vi "Autonomous Independent.vi"   [LabVIEW 2015]
doc: "This VI is called when autonomous begins, and will automatically be terminated when autonomous ends. You can carry out timed or sensor driven robot movement independently without needing to return to the caller."
uses:
  <vilib>/Rock Robotics/WPI/Utilities/WPI_GetSetVariantRefNum.vi
  <vilib>/Rock Robotics/Network Tables/NT Read String.vi
  <vilib>/Rock Robotics/Network Tables/NT Read Number.vi
  <vilib>/Rock Robotics/Network Tables/NT Write Numeric Array.vi
  <vilib>/Rock Robotics/Network Tables/NT Read Boolean.vi
panel:
  # "Be sure to right-click and choose Data Operations>>Make Current Value default if you want to save the array values with the VI"
types:
  T1 = typedef "WPI_JoystickDevRef.ctl" = cluster{"Device":T2}
  T2 = typedef "WPI_JoystickDeviceEnum.ctl" = enum16{"USB 0", "USB 1", "USB 2", "USB 3", "USB 4", "USB 5"}
  T3 = typedef "WPI_EncoderDevRef.ctl" = cluster{"DevStatus":errorcluster, "EncoderIndex":T4, "CounterIndex":T5, "DistancePerCount":dbl, "Decoding Type":T6}
  T4 = typedef "FPGA_EncoderIdx.ctl" = enum8{"Enc 0", "Enc 1", "Enc 2", "Enc 3", "Enc 4", "Enc 5", "Enc 6", "Enc 7", "Invalid"}
  T5 = typedef "FPGA_CounterCtrSystemIndex.ctl" = enum8{"Ctr 0", "Ctr 1", "Ctr 2", "Ctr 3", "Ctr 4", "Ctr 5", "Ctr 6", "Ctr 7", "Invalid"}
  T6 = typedef "WPI_EncoderType.ctl" = enum16{"1x", "2x", "4x"}
  T7 = typedef "WPI_MotorControlDeviceRef.ctl" = cluster{"DeviceStatus":errorcluster, "Type":T8, "PWM":cluster{"PWM Channel":T9, "DeadBand":T10}, "CAN":cluster{"Device Number":u8, "Control Mode":T11, "Semaphore":T12, "Max Vout":dbl, "TalonSRX Control Mode":T13}, "Invert":bool}
  T8 = typedef "WPI_MotorControlType.ctl" = enum16{"PWM", "CAN", "CANTalonSRX"}
  T9 = typedef "FPGA_DIOPWMChannel.ctl" = enum8{"PWM 0", "PWM 1", "PWM 2", "PWM 3", "PWM 4", "PWM 5", "PWM 6", "PWM 7", "PWM 8", "PWM 9", "PWM MXP 0", "PWM MXP 1", "PWM MXP 2", "PWM MXP 3", "PWM MXP 4", "PWM MXP 5", "PWM MXP 6", "PWM MXP 7", "PWM MXP 8", "PWM MXP 9", "Invalid"}
  T10 = typedef "WPI_PWMDeadband.ctl" = cluster{"Name":string, "maxPositivePwm":i32, "minPositivePwm":i32, "centerPwm":i32, "maxNegativePwm":i32, "minNegativePwm":i32, "angularRange":u16}
  T11 = typedef "WPI_CANJaguar_ControlMode.ctl" = enum8{"Percent VBus", "Current", "Speed", "Position", "Voltage"}
  T12 = typedef "Semaphore RefNum" = refnum<k1>
  T13 = typedef "WPI_CANTalonSRX_APIControlMode.ctl" = enum8{"Percent VBus", "Speed", "Position", "Slave", "Unchanged / Invalid", "Voltage Compensation", "Current", "Motion Profile"}
  T14 = typedef "WPI_GyroDevRef.ctl" = cluster{"DevStatus":errorcluster, "Analog Channel":T15, "Offset":dbl, "Gain (VoltsPerDegree/Second)":dbl, "Gyro Type":enum16{"Analog", "XRS450"}, "Handle":i32, "SPI Bus":T16, "Device Found":bool, "Sample Rate":dbl, "Calibrate On Open":bool}
  T15 = typedef "FPGA_AIChannel.ctl" = enum8{"AI 0", "AI 1", "AI 2", "AI 3", "AI MXP 0", "AI MXP 1", "AI MXP 2", "AI MXP 3", "Invalid"}
  T16 = typedef "spi_bus.ctl" = enum16{"SPI On-Board, CS0", "SPI On-Board, CS1", "SPI On-Board, CS2", "SPI On-Board, CS3", "SPI MXP", "Invalid"}
  T17 = typedef "WPI_RobotDriveDevRef.ctl" = cluster{"DevStatus":errorcluster, "Motors[]":T7[], "Square Inputs":bool, "Max Output":dbl}
  T18 = typedef "WPI_DigitalInputDevRef.ctl" = cluster{"DevStatus":errorcluster, "DIO Channel":T19}
  T19 = typedef "FPGA_DIOChannel.ctl" = enum8{"DIO 0", "DIO 1", "DIO 2", "DIO 3", "DIO 4", "DIO 5", "DIO 6", "DIO 7", "DIO 8", "DIO 9", "DIO MXP 0", "DIO MXP 1", "DIO MXP 2", "DIO MXP 3", "DIO MXP 4", "DIO MXP 5", "DIO MXP 6", "DIO MXP 7", "DIO MXP 8", "DIO MXP 9", "DIO MXP 10", "DIO MXP 11", "DIO MXP 12", "DIO MXP 13", "DIO MXP 14", "DIO MXP 15", "Invalid"}
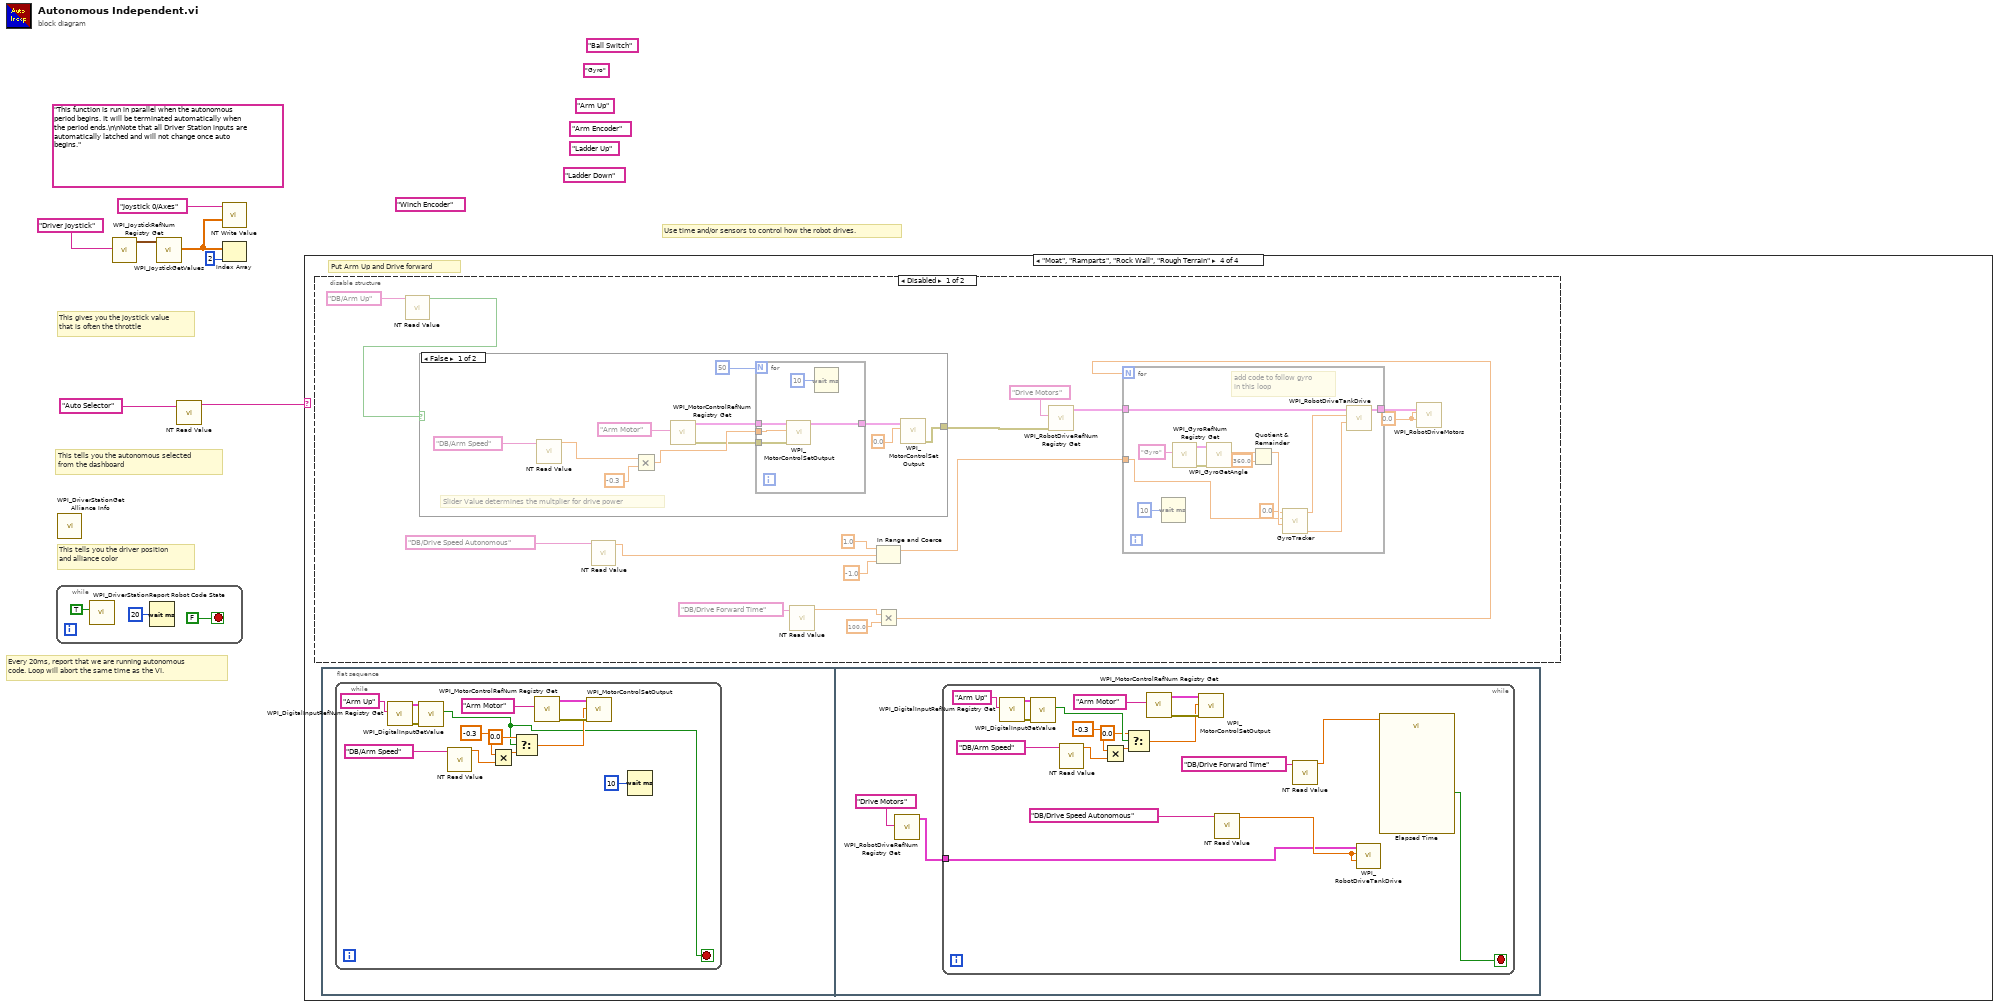
[diagram p0: block diagram]
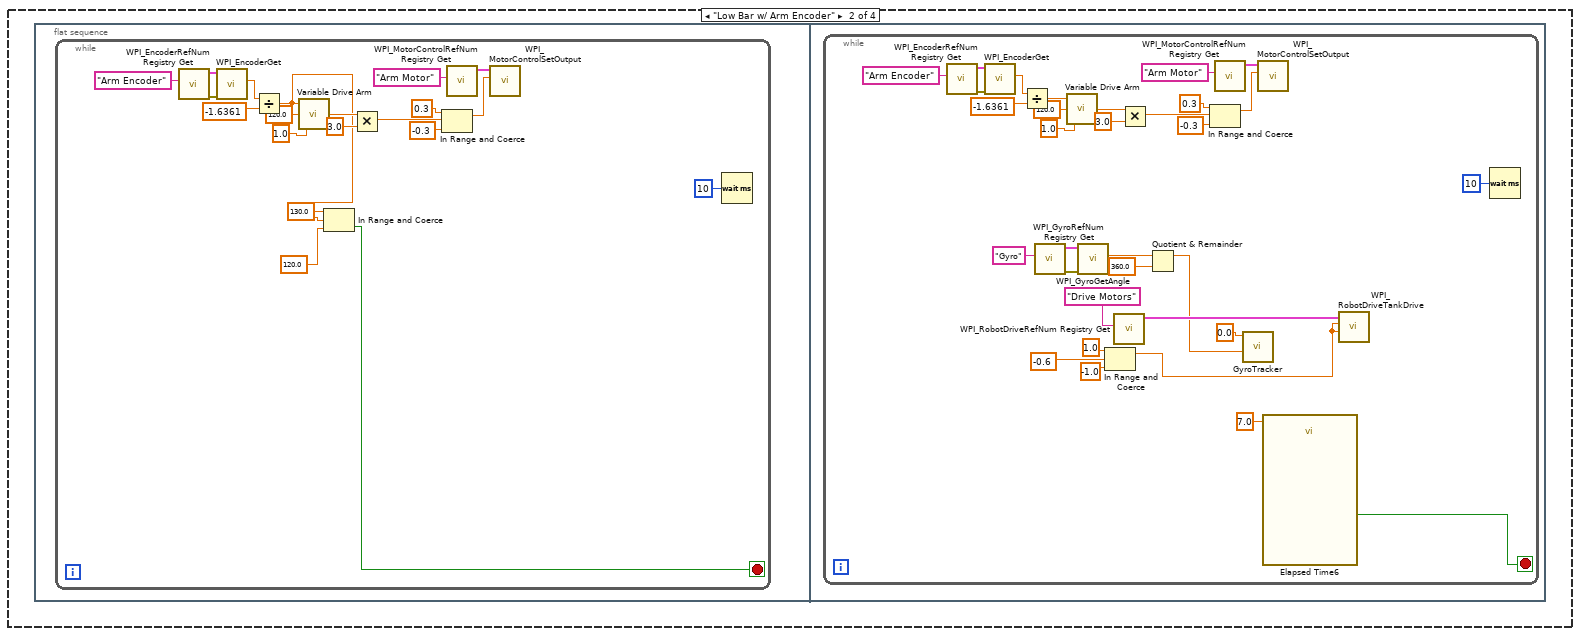
[diagram p3: hidden frame]
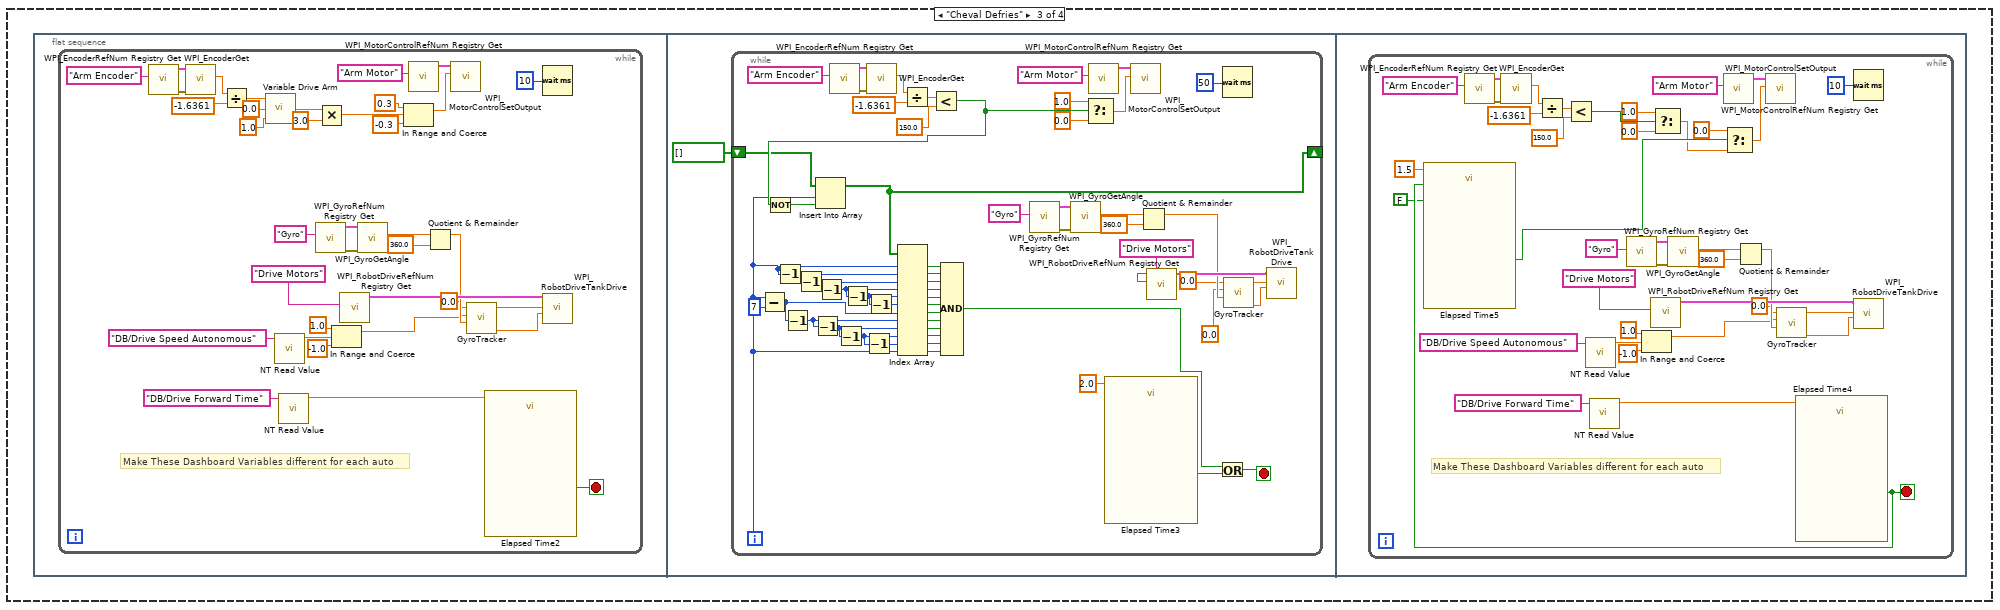
[diagram p4: hidden frame]
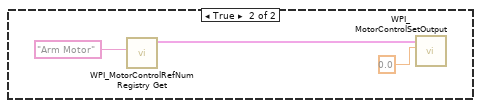
[diagram p5: hidden frame]
diagram:
  (unwired) "Arm Up" ("refnum name")
  (unwired) "Winch Encoder" ("refnum name")
  (unwired) "Ladder Down" ("refnum name")
  (unwired) "Ladder Up" ("refnum name")
  (unwired) "Arm Encoder" ("refnum name")
  (unwired) "Ball Switch" ("refnum name")
  (unwired) "Gyro" ("refnum name")
  (unwired) "This function is run in parallel when the autonomous period begins. It will be terminated automatically when the period ends.\n\nNote that all Driver Station inputs are automatically latched and will not change once auto begins."
  # "This tells you the autonomous selected\nfrom the dashboard"
  # "Every 20ms, report that we are running autonomous\ncode. Loop will abort the same time as the VI."
  # "This gives you the joystick value\nthat is often the throttle"
  # "Use time and/or sensors to control how the robot drives."
  # "This tells you the driver position\nand alliance color"
  n1 = while {
    stop <- FALSE stop-if-true
    n2 = call <vilib>:"WPI_DriverStationReport Robot Code State.vi"("Autonomous"=TRUE) -> ()  [unwired: 10 in, 1 out]
    n3 = Wait (ms)(milliseconds to wait=u32 20) -> ()  [unwired: 1 out]
  }
  n4 = call <vilib>:"WPI_DriverStationGet Alliance Info.vi"() -> ()  [unwired: 12 out]
  n5 = call <vilib>:"WPI_JoystickRefNum Registry Get.vi"("refnum name"="Driver Joystick") -> ("JoystickDevRef"=w6:T1)  [unwired: 1 in, 9 out]
  n6 = call <vilib>:"WPI_JoystickGetValues.vi"("JoystickDevRef"=w6) -> ("Axes"=w2:dbl[])  [unwired: 6 in, 4 out]
  n7 = call-poly <vilib>:"NT Read Value.vi"("Name"="Auto Selector") -> ("String"=w3:string)  [unwired: 9 in, 1 out]
  n8 = call-poly <vilib>:"NT Write Value.vi"("Numeric Array"=w2, "Name"="Joystick 0/Axes") -> ()  [unwired: 9 in, 1 out]
  n9 = Index Array(array=w2, index=2) -> ()  [unwired: 1 out]
  n10 = case shown="\"Moat\", \"Ramparts\", \"Rock Wall\", \"Rough Terrain\"" w3 {
    frame Default {
      # "You can put your main auto here, or you can right-click on the case and make any\nother frame be the default case."
      # "This is the frame that will execute if no selection is made, or if it is not recognized"
    }
    frame "Low Bar w/ Arm Encoder" {
      n11 = flat-sequence {
        frame #0 {
          n12 = while {
            stop <- w11 stop-if-true
            n13 = call <vilib>:"WPI_EncoderRefNum Registry Get.vi"("refnum name"="Arm Encoder") -> ("error out"=w24:errorcluster, "EncoderDevRef"=w25:T3)  [unwired: 9 in]
            n14 = call <vilib>:"WPI_EncoderGet.vi"("error in (no error)"=w24, "EncoderDevRef"=w25) -> ("Distance"=w26:dbl)  [unwired: 4 in, 5 out]
            n15 = Divide(x=w26, y=-1.6361 ("Arm Calibration")) -> (x/y=w14:dbl)
            n16 = call "Variable Drive Arm.vi"("Max Speed"=1.0, "Wanted Angle"=120.0, "Encoder"=w14) -> ("Motor Controller"=w18:dbl)
            n17 = In Range and Coerce(upper limit=130.0, x=w14, lower limit=120.0) -> (In Range?=w11:bool)  [unwired: 1 out]
            n18 = Multiply(x=w18, y=3.0) -> (x*y=w16:dbl)
            n19 = In Range and Coerce(upper limit=0.3, x=w16, lower limit=-0.3) -> (coerced(x)=w20:dbl)  [unwired: 1 out]
            n20 = call <vilib>:"WPI_MotorControlRefNum Registry Get.vi"("refnum name"="Arm Motor") -> ("MotorControlDevRef"=w21:T7)  [unwired: 9 in, 1 out]
            n21 = call <vilib>:"WPI_MotorControlSetOutput.vi"("Output"=w20, "MotorControlDevRef"=w21) -> ()  [unwired: 7 in, 3 out]
            n22 = Wait (ms)(milliseconds to wait=u32 10) -> ()  [unwired: 1 out]
          }
        }
        frame #1 {
          n23 = while {
            stop <- w62 stop-if-true
            n24 = call <vilib>:"WPI_EncoderRefNum Registry Get.vi"("refnum name"="Arm Encoder") -> ("error out"=w55:errorcluster, "EncoderDevRef"=w56:T3)  [unwired: 9 in]
            n25 = call <vilib>:"WPI_EncoderGet.vi"("error in (no error)"=w55, "EncoderDevRef"=w56) -> ("Distance"=w57:dbl)  [unwired: 4 in, 5 out]
            n26 = Divide(x=w57, y=-1.6361 ("Arm Calibration")) -> (x/y=w54:dbl)
            n27 = call <vilib>:"WPI_GyroRefNum Registry Get.vi"("refnum name"="Gyro") -> ("error out"=w36:errorcluster, "GyroDevRef"=w37:T14)  [unwired: 9 in]
            n28 = call "Variable Drive Arm.vi"("Max Speed"=1.0, "Wanted Angle"=120.0, "Encoder"=w54) -> ("Motor Controller"=w47:dbl)
            n29 = call <vilib>:"WPI_GyroGetAngle.vi"("error in"=w36, "GyroDevRef"=w37) -> ("Angle"=w39:dbl)  [unwired: 5 in, 4 out]
            n30 = In Range and Coerce(upper limit=1.0, x=-0.6, lower limit=-1.0) -> (coerced(x)=w33:dbl)  [unwired: 1 out]
            n31 = call <vilib>:"WPI_RobotDriveRefNum Registry Get.vi"("refnum name"="Drive Motors") -> ("RobotDriveDevRef"=w44:T17)  [unwired: 1 in, 9 out]
            n32 = Multiply(x=w47, y=3.0) -> (x*y=w45:dbl)
            n33 = Quotient & Remainder(x=w39, y=360.0) -> (x-y*floor(x/y)=w35:dbl)  [unwired: 1 out]
            n34 = In Range and Coerce(upper limit=0.3, x=w45, lower limit=-0.3) -> (coerced(x)=w50:dbl)  [unwired: 1 out]
            n35 = call <vilib>:"WPI_MotorControlRefNum Registry Get.vi"("refnum name"="Arm Motor") -> ("MotorControlDevRef"=w51:T7)  [unwired: 9 in, 1 out]
            n36 = call "GyroTracker.vi"("Gyro Angle"=w35, "Target Direction (degrees)"=0.0) -> ()  [unwired: 8 in, 2 out]
            n37 = call <vilib>:"WPI_MotorControlSetOutput.vi"("Output"=w50, "MotorControlDevRef"=w51) -> ()  [unwired: 7 in, 3 out]
            n38 = call "Elapsed Time6"("Time Target (s)"=7.0) -> ("Time has Elapsed"=w62:bool)  [unwired: 11 in, 7 out]
            n39 = call <vilib>:"WPI_RobotDriveTankDrive.vi"("Right axis value"=w33, "Left axis value"=w33, "RobotDriveDevRef"=w44) -> ()  [unwired: 6 in, 3 out]
            n40 = Wait (ms)(milliseconds to wait=u32 10) -> ()  [unwired: 1 out]
          }
        }
      }
    }
    frame "Cheval Defries" {
      n41 = flat-sequence {
        frame #0 {
          n42 = while {
            stop <- w98 stop-if-true
            # "Make These Dashboard Variables different for each auto"
            n43 = call <vilib>:"WPI_EncoderRefNum Registry Get.vi"("refnum name"="Arm Encoder") -> ("error out"=w91:errorcluster, "EncoderDevRef"=w92:T3)  [unwired: 9 in]
            n44 = call <vilib>:"WPI_EncoderGet.vi"("error in (no error)"=w91, "EncoderDevRef"=w92) -> ("Distance"=w93:dbl)  [unwired: 4 in, 5 out]
            n45 = Divide(x=w93, y=-1.6361 ("Arm Calibration")) -> (x/y=w90:dbl)
            n46 = call "Variable Drive Arm.vi"("Max Speed"=1.0, "Wanted Angle"=0.0, "Encoder"=w90) -> ("Motor Controller"=w83:dbl)
            n47 = call-poly <vilib>:"NT Read Value.vi"("Name"="DB/Drive Speed Autonomous") -> ("Numeric"=w77:dbl)  [unwired: 9 in, 1 out]
            n48 = call-poly <vilib>:"NT Read Value.vi"("Name"="DB/Drive Forward Time") -> ("Numeric"=w75:dbl)  [unwired: 9 in, 1 out]
            n49 = call <vilib>:"WPI_GyroRefNum Registry Get.vi"("refnum name"="Gyro") -> ("error out"=w66:errorcluster, "GyroDevRef"=w67:T14)  [unwired: 9 in]
            n50 = Multiply(x=w83, y=3.0) -> (x*y=w81:dbl)
            n51 = In Range and Coerce(upper limit=1.0, x=w77, lower limit=-1.0) -> (coerced(x)=w63:dbl)  [unwired: 1 out]
            n52 = call <vilib>:"WPI_RobotDriveRefNum Registry Get.vi"("refnum name"="Drive Motors") -> ("RobotDriveDevRef"=w73:T17)  [unwired: 1 in, 9 out]
            n53 = call <vilib>:"WPI_GyroGetAngle.vi"("error in"=w66, "GyroDevRef"=w67) -> ("Angle"=w69:dbl)  [unwired: 5 in, 4 out]
            n54 = In Range and Coerce(upper limit=0.3, x=w81, lower limit=-0.3) -> (coerced(x)=w86:dbl)  [unwired: 1 out]
            n55 = call <vilib>:"WPI_MotorControlRefNum Registry Get.vi"("refnum name"="Arm Motor") -> ("MotorControlDevRef"=w87:T7)  [unwired: 9 in, 1 out]
            n56 = Quotient & Remainder(x=w69, y=360.0) -> (x-y*floor(x/y)=w65:dbl)  [unwired: 1 out]
            n57 = call <vilib>:"WPI_MotorControlSetOutput.vi"("Output"=w86, "MotorControlDevRef"=w87) -> ()  [unwired: 7 in, 3 out]
            n58 = call "GyroTracker.vi"("Gyro Angle"=w65, "Target Speed"=w63, "Target Direction (degrees)"=0.0) -> ("Right Wheel Speed"=w71:dbl, "Left Wheel Speed"=w72:dbl)  [unwired: 7 in]
            n59 = call "Elapsed Time2"("Time Target (s)"=w75) -> ("Time has Elapsed"=w98:bool)  [unwired: 11 in, 7 out]
            n60 = Wait (ms)(milliseconds to wait=u32 10) -> ()  [unwired: 1 out]
            n61 = call <vilib>:"WPI_RobotDriveTankDrive.vi"("Right axis value"=w71, "Left axis value"=w72, "RobotDriveDevRef"=w73) -> ()  [unwired: 6 in, 3 out]
          }
        }
        frame #1 {
          n62 = while {
            shift-right: [w104] -> _
            shift-left: bool[] [] -> [w105]
            i -> [w103]
            stop <- w108 stop-if-true
            n63 = Subtract(x=w103, y=7) -> (x-y=w125:i32)
            n64 = Decrement(x=w103) -> (x-1=w128:i32)
            n65 = Decrement(x=w125) -> (x-1=w124:i32)
            n66 = Decrement(x=w128) -> (x-1=w130:i32)
            n67 = Decrement(x=w124) -> (x-1=w123:i32)
            n68 = Decrement(x=w130) -> (x-1=w132:i32)
            n69 = call <vilib>:"WPI_EncoderRefNum Registry Get.vi"("refnum name"="Arm Encoder") -> ("error out"=w138:errorcluster, "EncoderDevRef"=w139:T3)  [unwired: 9 in]
            n70 = Decrement(x=w123) -> (x-1=w121:i32)
            n71 = Decrement(x=w132) -> (x-1=w129:i32)
            n72 = Decrement(x=w121) -> (x-1=w122:i32)
            n73 = call <vilib>:"WPI_EncoderGet.vi"("error in (no error)"=w138, "EncoderDevRef"=w139) -> ("Distance"=w140:dbl)  [unwired: 4 in, 5 out]
            n74 = Decrement(x=w129) -> (x-1=w131:i32)
            n75 = Divide(x=w140, y=-1.6361 ("Arm Calibration")) -> (x/y=w133:dbl)
            n76 = Less?(x=w133, y=150.0) -> (x < y?=w106:bool)
            n77 = Not(x=w106) -> (.not. x?=w100:bool)
            n78 = Insert Into Array(array=w105, index=w103, new element=w100) -> (w104:bool[])
            n79 = Index Array(array=w104, index #1=w103, index #2=w128, index #3=w130, index #4=w132, index #5=w129, index #6=w131, index #7=w125, index #8=w124, index #9=w123, index #10=w121, index #11=w122, index #12=w103) -> (element #1=w120:bool, element #2=w119:bool, element #3=w118:bool, element #4=w117:bool, element #5=w116:bool, element #6=w115:bool, element #7=w114:bool, element #8=w113:bool, element #9=w112:bool, element #10=w111:bool, element #11=w110:bool, element #12=w102:bool)
            n80 = Compound Arithmetic op=AND(w120, w119, w118, w117, w116, w115, w114, w113, w112, w111, w110, w102) -> (w101:bool)
            n81 = call <vilib>:"WPI_GyroRefNum Registry Get.vi"("refnum name"="Gyro") -> ("error out"=w146:errorcluster, "GyroDevRef"=w147:T14)  [unwired: 9 in]
            n82 = call <vilib>:"WPI_GyroGetAngle.vi"("error in"=w146, "GyroDevRef"=w147) -> ("Angle"=w149:dbl)  [unwired: 5 in, 4 out]
            n83 = Select(t=1.0, s=w106, f=0.0) -> (s? t:f=w136:dbl)
            n84 = call <vilib>:"WPI_MotorControlRefNum Registry Get.vi"("refnum name"="Arm Motor") -> ("MotorControlDevRef"=w155:T7)  [unwired: 9 in, 1 out]
            n85 = call "Elapsed Time3"("Time Target (s)"=2.0) -> ("Time has Elapsed"=w109:bool)  [unwired: 11 in, 7 out]
            n86 = call <vilib>:"WPI_MotorControlSetOutput.vi"("Output"=w136, "MotorControlDevRef"=w155) -> ()  [unwired: 7 in, 3 out]
            n87 = Quotient & Remainder(x=w149, y=360.0) -> (x-y*floor(x/y)=w145:dbl)  [unwired: 1 out]
            n88 = call <vilib>:"WPI_RobotDriveRefNum Registry Get.vi"("refnum name"="Drive Motors") -> ("RobotDriveDevRef"=w152:T17)  [unwired: 1 in, 9 out]
            n89 = Or(x=w101, y=w109) -> (x .or. y?=w108:bool)
            n90 = Wait (ms)(milliseconds to wait=u32 50) -> ()  [unwired: 1 out]
            n91 = call "GyroTracker.vi"("Gyro Angle"=w145, "Target Speed"=0.0, "Target Direction (degrees)"=0.0) -> ("Right Wheel Speed"=w127:dbl, "Left Wheel Speed"=w151:dbl)  [unwired: 7 in]
            n92 = call <vilib>:"WPI_RobotDriveTankDrive.vi"("Right axis value"=w127, "Left axis value"=w151, "RobotDriveDevRef"=w152) -> ()  [unwired: 6 in, 3 out]
          }
        }
        frame #2 {
          n93 = while {
            stop <- w162 stop-if-true
            # "Make These Dashboard Variables different for each auto"
            n94 = call <vilib>:"WPI_EncoderRefNum Registry Get.vi"("refnum name"="Arm Encoder") -> ("error out"=w169:errorcluster, "EncoderDevRef"=w170:T3)  [unwired: 9 in]
            n95 = call <vilib>:"WPI_EncoderGet.vi"("error in (no error)"=w169, "EncoderDevRef"=w170) -> ("Distance"=w171:dbl)  [unwired: 4 in, 5 out]
            n96 = Divide(x=w171, y=-1.6361 ("Arm Calibration")) -> (x/y=w165:dbl)
            n97 = Less?(x=w165, y=150.0) -> (x < y?=w164:bool)
            n98 = call-poly <vilib>:"NT Read Value.vi"("Name"="DB/Drive Speed Autonomous") -> ("Numeric"=w190:dbl)  [unwired: 9 in, 1 out]
            n99 = call-poly <vilib>:"NT Read Value.vi"("Name"="DB/Drive Forward Time") -> ("Numeric"=w188:dbl)  [unwired: 9 in, 1 out]
            n100 = call <vilib>:"WPI_GyroRefNum Registry Get.vi"("refnum name"="Gyro") -> ("error out"=w179:errorcluster, "GyroDevRef"=w180:T14)  [unwired: 9 in]
            n101 = In Range and Coerce(upper limit=1.0, x=w190, lower limit=-1.0) -> (coerced(x)=w176:dbl)  [unwired: 1 out]
            n102 = call <vilib>:"WPI_RobotDriveRefNum Registry Get.vi"("refnum name"="Drive Motors") -> ("RobotDriveDevRef"=w186:T17)  [unwired: 1 in, 9 out]
            n103 = Select(t=1.0, s=w164, f=0.0) -> (s? t:f=w157:dbl)
            n104 = call <vilib>:"WPI_GyroGetAngle.vi"("error in"=w179, "GyroDevRef"=w180) -> ("Angle"=w182:dbl)  [unwired: 5 in, 4 out]
            n105 = call <vilib>:"WPI_MotorControlRefNum Registry Get.vi"("refnum name"="Arm Motor") -> ("MotorControlDevRef"=w174:T7)  [unwired: 9 in, 1 out]
            n106 = Quotient & Remainder(x=w182, y=360.0) -> (x-y*floor(x/y)=w178:dbl)  [unwired: 1 out]
            n107 = call "GyroTracker.vi"("Gyro Angle"=w178, "Target Speed"=w176, "Target Direction (degrees)"=0.0) -> ("Right Wheel Speed"=w184:dbl, "Left Wheel Speed"=w185:dbl)  [unwired: 7 in]
            n108 = call "Elapsed Time4"("Time Target (s)"=w188) -> ("Time has Elapsed"=w162:bool)  [unwired: 11 in, 7 out]
            n109 = call "Elapsed Time5"("Time Target (s)"=1.5, "Reset"=w162, "Auto Reset"=FALSE) -> ("Time has Elapsed"=w159:bool)  [unwired: 9 in, 7 out]
            n110 = Select(t=0.0, s=w159, f=w157) -> (s? t:f=w160:dbl)
            n111 = call <vilib>:"WPI_MotorControlSetOutput.vi"("Output"=w160, "MotorControlDevRef"=w174) -> ()  [unwired: 7 in, 3 out]
            n112 = Wait (ms)(milliseconds to wait=u32 10) -> ()  [unwired: 1 out]
            n113 = call <vilib>:"WPI_RobotDriveTankDrive.vi"("Right axis value"=w184, "Left axis value"=w185, "RobotDriveDevRef"=w186) -> ()  [unwired: 6 in, 3 out]
          }
        }
      }
    }
    frame "Moat", "Ramparts", "Rock Wall", "Rough Terrain" {
      # "Put Arm Up and Drive forward"
      n114 = disable-structure shown="Disabled" {
        frame Disabled {
          w207 = 0.0 ("Y axis value")
          n115 = call-poly <vilib>:"NT Read Value.vi"("Name"="DB/Arm Up") -> ("Boolean"=w200:bool)  [unwired: 9 in, 1 out]
          n116 = case shown="False" w200 {
            tunnel: [w211 _] -> w201
            frame False {
              # "Slider Value determines the multplier for drive power"
              n117 = call-poly <vilib>:"NT Read Value.vi"("Name"="DB/Arm Speed") -> ("Numeric"=w216:dbl)  [unwired: 9 in, 1 out]
              n118 = Multiply(x=w216, y=-0.3) -> (x*y=w221:dbl)
              n119 = call <vilib>:"WPI_MotorControlRefNum Registry Get.vi"("refnum name"="Arm Motor") -> ("error out"=w220:errorcluster, "MotorControlDevRef"=w219:T7)  [unwired: 9 in]
              n120 = for {
                N: 50 -> [_]
                tunnel: w219 -> [w225]
                tunnel: w220 -> [w224]
                tunnel: w221 -> [w223]
                tunnel: [w222] -> w212
                n121 = call <vilib>:"WPI_MotorControlSetOutput.vi"("error in (no error)"=w224, "Output"=w223, "MotorControlDevRef"=w225) -> ("MotorControlDevRef"=w222:T7)  [unwired: 6 in, 2 out]
                n122 = Wait (ms)(milliseconds to wait=u32 10) -> ()  [unwired: 1 out]
              }
              n123 = call <vilib>:"WPI_MotorControlSetOutput.vi"("Output"=0.0, "MotorControlDevRef"=w212) -> ("error out"=w211:errorcluster)  [unwired: 7 in, 2 out]
            }
            frame True {
              n124 = call <vilib>:"WPI_MotorControlRefNum Registry Get.vi"("refnum name"="Arm Motor") -> ("MotorControlDevRef"=w228:T7)  [unwired: 9 in, 1 out]
              n125 = call <vilib>:"WPI_MotorControlSetOutput.vi"("Output"=0.0, "MotorControlDevRef"=w228) -> ()  [unwired: 7 in, 3 out]
            }
          }
          n126 = call-poly <vilib>:"NT Read Value.vi"("Name"="DB/Drive Speed Autonomous") -> ("Numeric"=w205:dbl)  [unwired: 9 in, 1 out]
          n127 = call-poly <vilib>:"NT Read Value.vi"("Name"="DB/Drive Forward Time") -> ("Numeric"=w196:dbl)  [unwired: 9 in, 1 out]
          n128 = In Range and Coerce(upper limit=1.0, x=w205, lower limit=-1.0) -> (coerced(x)=w199:dbl)  [unwired: 1 out]
          n129 = Multiply(x=w196, y=100.0) -> (x*y=w198:dbl)
          n130 = call <vilib>:"WPI_RobotDriveRefNum Registry Get.vi"("error in (no error)"=w201, "refnum name"="Drive Motors") -> ("RobotDriveDevRef"=w209:T17)  [unwired: 9 out]
          n131 = for {
            N: w198 -> [_]
            tunnel: w209 -> [w232]
            tunnel: w199 -> [w230]
            tunnel: [w231] -> w208
            # "add code to follow gyro\nin this loop"
            n132 = Wait (ms)(milliseconds to wait=u32 10) -> ()  [unwired: 1 out]
            n133 = call <vilib>:"WPI_GyroRefNum Registry Get.vi"("refnum name"="Gyro") -> ("error out"=w235:errorcluster, "GyroDevRef"=w236:T14)  [unwired: 9 in]
            n134 = call <vilib>:"WPI_GyroGetAngle.vi"("error in"=w235, "GyroDevRef"=w236) -> ("Angle"=w238:dbl)  [unwired: 5 in, 4 out]
            n135 = Quotient & Remainder(x=w238, y=360.0) -> (x-y*floor(x/y)=w234:dbl)  [unwired: 1 out]
            n136 = call "GyroTracker.vi"("Gyro Angle"=w234, "Target Speed"=w230, "Target Direction (degrees)"=0.0) -> ("Right Wheel Speed"=w240:dbl, "Left Wheel Speed"=w241:dbl)  [unwired: 7 in]
            n137 = call <vilib>:"WPI_RobotDriveTankDrive.vi"("Right axis value"=w240, "Left axis value"=w241, "RobotDriveDevRef"=w232) -> ("RobotDriveDevRef"=w231:T17)  [unwired: 6 in, 2 out]
          }
          n138 = call <vilib>:"WPI_RobotDriveMotors.vi"("RightSpeed"=w207, "LeftSpeed"=w207, "RobotDriveDevRef"=w208) -> ()  [unwired: 6 in, 3 out]
        }
        frame Enabled {
        }
      }
      n139 = flat-sequence {
        frame #0 {
          n140 = while {
            stop <- w244 stop-if-true
            n141 = call <vilib>:"WPI_DigitalInputRefNum Registry Get.vi"("refnum name"="Arm Up") -> ("error out"=w255:errorcluster, "DigitalInputDevRef"=w254:T18)  [unwired: 9 in]
            n142 = call <vilib>:"WPI_DigitalInputGetValue.vi"("error in (no error)"=w255, "DigitalInputDevRef"=w254) -> ("Value"=w244:bool)  [unwired: 7 in, 2 out]
            n143 = call-poly <vilib>:"NT Read Value.vi"("Name"="DB/Arm Speed") -> ("Numeric"=w249:dbl)  [unwired: 9 in, 1 out]
            n144 = Multiply(x=-0.3 ("Numeric"), y=w249) -> (x*y=w248:dbl)
            n145 = Select(t=0.0, s=w244, f=w248) -> (s? t:f=w245:dbl)
            n146 = call <vilib>:"WPI_MotorControlRefNum Registry Get.vi"("refnum name"="Arm Motor") -> ("error out"=w251:errorcluster, "MotorControlDevRef"=w252:T7)  [unwired: 9 in]
            n147 = call <vilib>:"WPI_MotorControlSetOutput.vi"("error in (no error)"=w251, "Output"=w245, "MotorControlDevRef"=w252) -> ()  [unwired: 6 in, 3 out]
            n148 = Wait (ms)(milliseconds to wait=u32 10) -> ()  [unwired: 1 out]
          }
        }
        frame #1 {
          n149 = call <vilib>:"WPI_RobotDriveRefNum Registry Get.vi"("refnum name"="Drive Motors") -> ("RobotDriveDevRef"=w257:T17)  [unwired: 1 in, 9 out]
          n150 = while {
            tunnel: w257 -> [w259]
            stop <- w261 stop-if-true
            n151 = call <vilib>:"WPI_DigitalInputRefNum Registry Get.vi"("refnum name"="Arm Up") -> ("error out"=w276:errorcluster, "DigitalInputDevRef"=w275:T18)  [unwired: 9 in]
            n152 = call <vilib>:"WPI_DigitalInputGetValue.vi"("error in (no error)"=w276, "DigitalInputDevRef"=w275) -> ("Value"=w267:bool)  [unwired: 7 in, 2 out]
            n153 = call-poly <vilib>:"NT Read Value.vi"("Name"="DB/Arm Speed") -> ("Numeric"=w270:dbl)  [unwired: 9 in, 1 out]
            n154 = Multiply(x=-0.3 ("Numeric"), y=w270) -> (x*y=w269:dbl)
            n155 = Select(t=0.0, s=w267, f=w269) -> (s? t:f=w265:dbl)
            n156 = call <vilib>:"WPI_MotorControlRefNum Registry Get.vi"("refnum name"="Arm Motor") -> ("error out"=w272:errorcluster, "MotorControlDevRef"=w273:T7)  [unwired: 9 in]
            n157 = call <vilib>:"WPI_MotorControlSetOutput.vi"("error in (no error)"=w272, "Output"=w265, "MotorControlDevRef"=w273) -> ()  [unwired: 6 in, 3 out]
            n158 = call-poly <vilib>:"NT Read Value.vi"("Name"="DB/Drive Speed Autonomous") -> ("Numeric"=w260:dbl)  [unwired: 9 in, 1 out]
            n159 = call-poly <vilib>:"NT Read Value.vi"("Name"="DB/Drive Forward Time") -> ("Numeric"=w262:dbl)  [unwired: 9 in, 1 out]
            n160 = call <vilib>:"WPI_RobotDriveTankDrive.vi"("Right axis value"=w260, "Left axis value"=w260, "RobotDriveDevRef"=w259) -> ()  [unwired: 6 in, 3 out]
            n161 = call "Elapsed Time"("Time Target (s)"=w262) -> ("Time has Elapsed"=w261:bool)  [unwired: 11 in, 7 out]
          }
        }
      }
    }
  }
